vi "SendAndGetData.vi"(0 "reference":refnum<class "VdRs232.lvclass">, 1 "CharacterToWrite":string, 2 "MatchPatternToIndicateCompleteResponse(Use default if not wired)":string, 3 "TimeOut(Use default if not wired)":i32=-1, 4 "numberOfBytes(-1=all)":i32=-1, 5 "error in (no error)":errorcluster, 8 "Don'tLockAccess(False)\nOnly use this is you've locked access yourself":bool) -> (14 "reference out":refnum<class "VdRs232.lvclass">, 15 "ResponseMessage":string, 16 "TimeOut":bool, 17 "Time(ms)":u32, 19 "error out":errorcluster)   [LabVIEW 2020, in "VdRs232.lvclass"]
doc: "SendAndGetData"
uses:
  VdRs232.lvclass
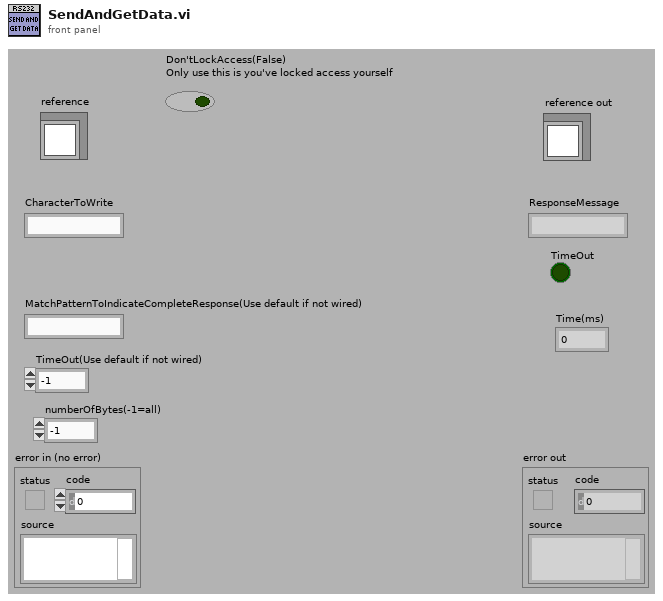
[diagram p1: front panel]
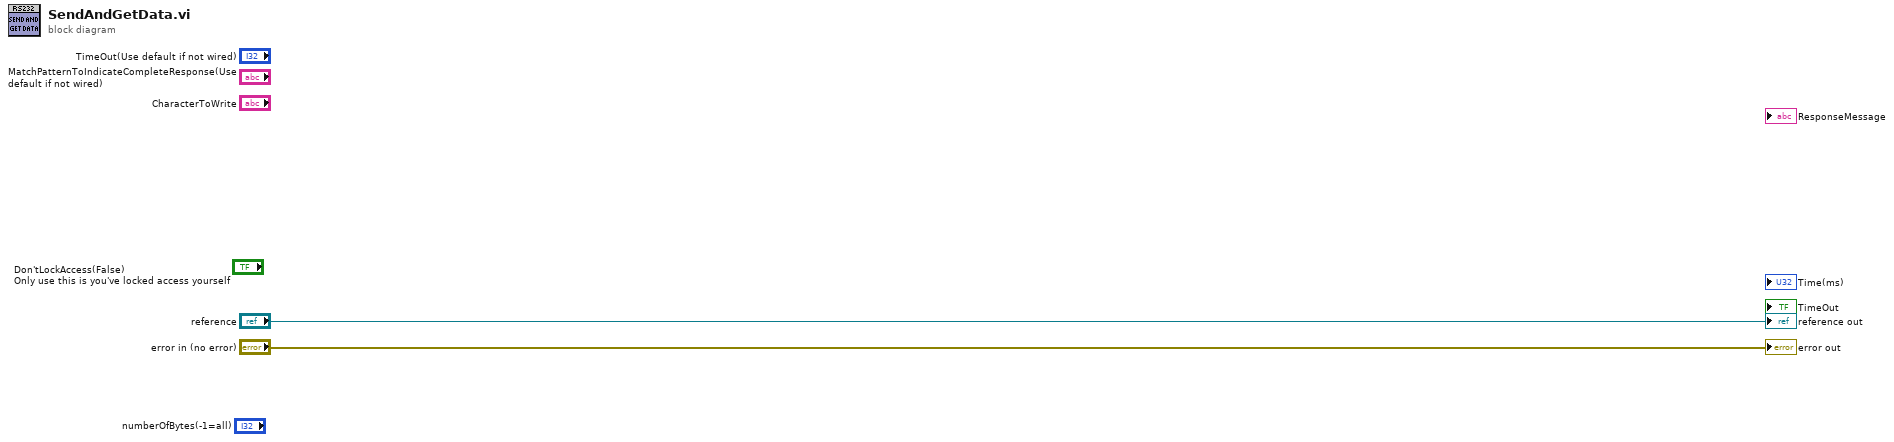
[diagram p0: block diagram]
diagram:
  "reference out" <- "reference"
  "error out" <- "error in (no error)"
